vi "disable.vi"(8 "error in (no error)":errorcluster, 11 "Tv in":refnum<class "Tv.lvclass">) -> (0 "error out":errorcluster, 3 "Tv out":refnum<class "Tv.lvclass">)   [LabVIEW 2017, in "Tv.lvclass"]
uses:
  Tv.lvclass
  Tv.lvclass/Tv.ctl
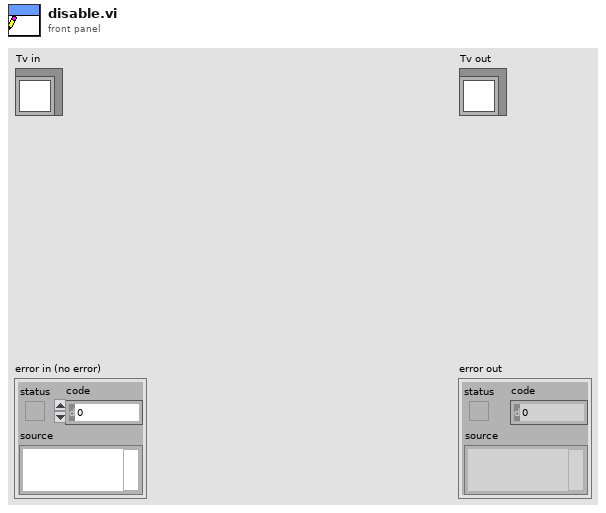
[diagram p1: front panel]
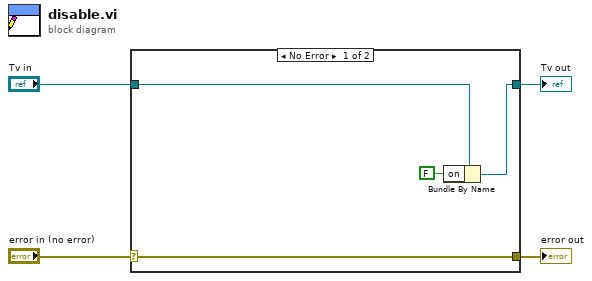
[diagram p0: block diagram]
diagram:
  n1 = case shown="No Error" "error in (no error)" {
    selector: "error in (no error)" -> [w8 w9]
    tunnel: [w8 w9] -> w3
    tunnel: [w6 w10] -> w1
    tunnel: "Tv in" -> [w7 w10]
    frame No Error {
      n2 = Bundle By Name(cluster=w7, "on"=FALSE) -> (w6:refnum<class "Tv.lvclass">)
    }
    frame Error {
    }
  }
  "error out" <- w3
  "Tv out" <- w1
